vi "Check Status.vi"(8 "error in (no error)":errorcluster, 11 "Wavelength Meter in":refnum<class "Wavelength Meter.lvclass">) -> (0 "error out":errorcluster, 1 "Status":string, 2 "Ready?":bool, 3 "Wavelength Meter out":refnum<class "Wavelength Meter.lvclass">)   [LabVIEW 2017, in "Wavelength Meter.lvclass"]
doc: "(Dynamic) Check if the instrument is powered on and update its member fields with the instrument's current status. Optionally return a text status message."
uses:
  Wavelength Meter.lvclass
  Wavelength Meter.lvclass/Wavelength Meter.ctl
  Utility Classes/Readable/Readable.lvclass
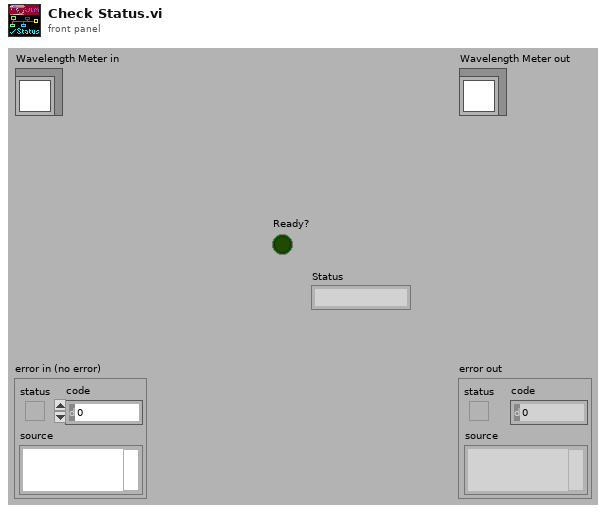
[diagram p1: front panel]
types:
  T1 = typedef "HighFinesse WS5.lvlib/Exposure Mode.ctl" = enum16{"manual", "automatic"}
  T2 = typedef "HighFinesse WS5.lvlib/Measurement Mode.ctl" = enum16{"Measurement off", "Adjustment mode", "Measurement mode"}
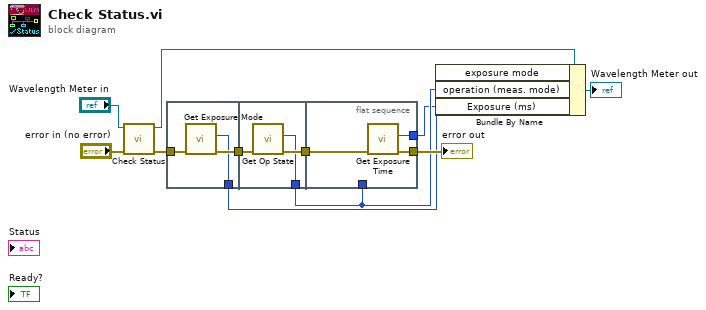
[diagram p0: block diagram]
diagram:
  n1 = call-parent "Check Status.vi"("error in (no error)"="error in (no error)", "Instrument in"="Wavelength Meter in") -> ("error out"=w9:errorcluster, "Instrument out"=w8:refnum<class "Wavelength Meter.lvclass">)  [unwired: 6 in, 2 out]
  n2 = flat-sequence {
    tunnel: w9 -> [w14]
    tunnel: [w13] -> w6
    tunnel: [w12] -> w4
    tunnel: w6 -> [w17]
    tunnel: [w16] -> w3
    tunnel: [w15] -> w2
    tunnel: w2 -> [_]
    tunnel: [w19] -> w5
    tunnel: w3 -> [w20]
    tunnel: [w18] -> w1
    frame #0 {
      n3 = call "Get Exposure Mode.vi"("error in (no error)"=w14) -> ("error out"=w13:errorcluster, "exposure mode"=w12:T1)  [unwired: 9 in]
    }
    frame #1 {
      n4 = call "Get Op State.vi"("error in (no error)"=w17) -> ("error out"=w16:errorcluster, "operation (meas. mode)"=w15:T2)  [unwired: 9 in]
    }
    frame #2 {
      n5 = call "Get Exposure Time.vi"("error in (no error)"=w20) -> ("error out"=w19:errorcluster, "Exposure (ms)"=w18:u16)  [unwired: 9 in]
    }
  }
  n6 = Bundle By Name(cluster=w8, "exposure mode"=w4, "operation (meas. mode)"=w2, "Exposure (ms)"=w1) -> (→"Wavelength Meter out":refnum<class "Wavelength Meter.lvclass">)
  "error out" <- w5
